vi "property.get.vi"   [LabVIEW 2020, in "asset.lvclass"]
uses:
  asset.lvclass
  asset.lvclass/asset.ctl
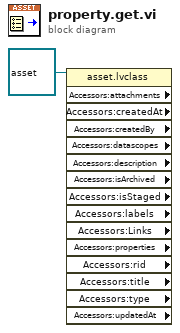
[diagram p0: block diagram]
diagram:
  n1 = property class="asset.lvclass" props=["Accessors:attachments", "Accessors:createdAt", "Accessors:createdBy", "Accessors:datascopes", "Accessors:description", "Accessors:isArchived", "Accessors:isStaged", "Accessors:labels", "Accessors:Links", "Accessors:properties", "Accessors:rid", "Accessors:title", "Accessors:type", "Accessors:updatedAt"](reference=refnum<class "asset.lvclass"> refnum ("asset.lvclass")) -> ()  [unwired: 1 in, 16 out]
